vi "Lab Panel V4.91.vi"() -> ()   [LabVIEW 2013] (continued)
                          tunnel: w2787 -> [w2790 _]
                          tunnel: w2786 -> [_ w2795]
                          tunnel: w2785 -> [w2788 _]
                          frame #0 {
                            n1476 = Build Array("T-RISE") -> (w2792:string[])
                            n1477 = Build Array(w2790) -> (w2791:dbl[])
                            n1478 = TDMS Write(0:w2788, 5:"TEST PASS", 7:w2792, 9:w2791) -> (15:w2794:errorcluster)  [unwired: 2 in, 3 out]
                            n1479 = local write "data file error"(w2794) -> ()
                          }
                          frame #1 {
                            n1480 = Bundle(cluster=w2795, "STATUS"="T-RISE PASS") -> (w2797:T4)  [unwired: 2 in]
                            n1481 = local write "RESULT LAB05-2"(TRUE) -> ()
                            n1482 = local write "DISP LAB05-2"(w2797) -> ()
                          }
                        }
                      }
                      frame False {
                      }
                    }
                  }
                }
              }
            }
          }
          frame #6 {
            # "end test & close test files"
            n1483 = local read "MAIL SETTINGS"() -> (w2803:T7)
            n1484 = Unbundle(w2803) -> ("OUT SERVER ADDRESS"=w2802:string, "FROM ACCOUNT"=w2801:string)  [unwired: 5 out]
            n1485 = stacked-sequence {
              tunnel: w2813 -> [_ _ _ _ _ _ _ _ _ _]
              tunnel: w2814 -> [_ _ _ _ _ _ _ _ _ _]
              tunnel: w2812 -> [_ _ _ _ _ _ _ _ _ _]
              tunnel: w2811 -> [_ _ _ _ _ _ _ _ _ _]
              tunnel: w2810 -> [_ _ _ _ _ _ _ _ _ _]
              tunnel: w2809 -> [_ _ _ _ _ _ _ _ _ _]
              tunnel: w2808 -> [_ _ _ _ _ _ _ _ _ _]
              tunnel: w2807 -> [_ _ _ _ _ _ _ _ _ _]
              tunnel: w2806 -> [_ _ _ _ _ _ _ _ _ _]
              tunnel: w2805 -> [_ _ _ _ _ _ _ _ _ _]
              tunnel: w2802 -> [w2818 w2870 w2918 w2965 w3012 w3059 w3106 w3153 w3200 w3247]
              tunnel: w2801 -> [w2817 w2869 w2917 w2964 w3011 w3058 w3105 w3152 w3199 w3246]
              tunnel: "Mail Test File To:" -> [w2816 w2868 w2916 w2963 w3010 w3057 w3104 w3151 w3198 w3245]
              tunnel: "Mail Test Fail" -> [w2815 w2867 w2915 w2962 w3009 w3056 w3103 w3150 w3197 w3244]
              frame #0 {
                # "LAB01-1"
                n1486 = local read "DISP LAB01-1"() -> (w2822:T4)
                n1487 = local read "run lab01-1"() -> (w2819:bool)
                n1488 = local read "TDMS LAB01-1"() -> (w2820:refnum<k34>)
                n1489 = Unbundle(w2822) -> ("CYCLE"=w2823:dbl, "STATUS"=w2821:string)  [unwired: 1 out]
                n1490 = case shown="True" w2819 {
                  tunnel: w2823 -> [_ w2829]
                  tunnel: w2822 -> [_ w2831]
                  tunnel: w2821 -> [_ w2828]
                  tunnel: w2820 -> [_ w2830]
                  tunnel: w2818 -> [_ w2827]
                  tunnel: w2817 -> [_ w2826]
                  tunnel: w2816 -> [_ w2825]
                  tunnel: w2815 -> [_ w2824]
                  frame False {
                  }
                  frame True {
                    n1491 = Not Equal?(x=w2828, y="RUN") -> (x != y?=w2832:bool)
                    n1492 = Greater?(x=w2829, y=2.0) -> (0:w2834:bool)
                    n1493 = And(x=w2834, y=w2832) -> (x .and. y?=w2833:bool)
                    n1494 = case shown="True" w2833 {
                      tunnel: w2831 -> [_ w2844]
                      tunnel: w2830 -> [_ w2843]
                      tunnel: w2829 -> [_ w2842]
                      tunnel: w2828 -> [_ w2841]
                      tunnel: w2827 -> [_ w2840]
                      tunnel: w2826 -> [_ w2839]
                      tunnel: w2825 -> [_ w2838]
                      tunnel: w2824 -> [_ w2837]
                      frame False {
                      }
                      frame True {
                        n1495 = stacked-sequence {
                          tunnel: w2844 -> [w2848 _ _]
                          tunnel: w2843 -> [_ w2850 _]
                          tunnel: w2842 -> [_ _ _]
                          tunnel: w2841 -> [_ _ w2856]
                          tunnel: w2840 -> [_ _ w2855]
                          tunnel: w2839 -> [_ _ w2854]
                          tunnel: w2838 -> [_ _ w2853]
                          tunnel: w2837 -> [_ _ w2852]
                          frame #0 {
                            w2845 = FALSE
                            n1496 = local write "mail control"("END") -> ()
                            n1497 = Bundle(cluster=w2848) -> (w2847:T4)  [unwired: 3 in]
                            n1498 = local write "DISP LAB01-1"(w2847) -> ()
                            n1499 = local write "O/I  LAB01-1"(w2845) -> ()
                            n1500 = local write "run lab01-1"(w2845) -> ()
                            n1501 = local write "RUN LAB01-1"(w2845) -> ()
                          }
                          frame #1 {
                            n1502 = TDMS Close(11:w2850) -> (0:w2849:errorcluster)  [unwired: 1 in, 1 out]
                            n1503 = local write "data file error"(w2849) -> ()
                          }
                          frame #2 {
                            n1504 = stacked-sequence {
                              tunnel: "LAB01-1" -> [w2858 w2860 _]
                              tunnel: w2856 -> [_ w2866 _]
                              tunnel: w2855 -> [_ w2865 _]
                              tunnel: w2854 -> [_ w2864 _]
                              tunnel: w2853 -> [_ w2863 _]
                              tunnel: w2852 -> [_ w2862 _]
                              frame #0 {
                                n1505 = call "sub vi - defrag tdms v1.vi"("panel id"=w2858) -> ("error out"=w2857:errorcluster)  [unwired: 10 in]
                                n1506 = local write "data file error"(w2857) -> ()
                              }
                              frame #1 {
                                n1507 = Bundle("STATUS"=w2866, "OUT SERVER ADDRESS"=w2865, "FROM ACCOUNT"=w2864, "Mail Test File To:"=w2863, "Mail Test Fail"=w2862) -> (w2859:T25)  [unwired: 1 in]
                                n1508 = call "Save data file (pass-fail) v5.vi"("Input Cluster"=w2859, "panel id"=w2860) -> ("network file save error"=w2861:errorcluster)  [unwired: 8 in, 1 out]
                                n1509 = local write "data file error"(w2861) -> ()
                              }
                              frame #2 {
                              }
                            }
                          }
                        }
                      }
                    }
                  }
                }
              }
              frame #1 {
                # "LAB01-2"
                n1510 = local read "run lab01-2"() -> (w2871:bool)
                n1511 = case shown="True" w2871 {
                  tunnel: w2870 -> [_ w2875]
                  tunnel: w2869 -> [_ w2874]
                  tunnel: w2868 -> [_ w2873]
                  tunnel: w2867 -> [_ w2872]
                  frame False {
                  }
                  frame True {
                    n1512 = local read "DISP LAB01-2"() -> (w2883:T4)
                    n1513 = local read "TDMS LAB01-2"() -> (w2882:refnum<k34>)
                    n1514 = Unbundle(w2883) -> ("CYCLE"=w2877:dbl, "STATUS"=w2876:string)  [unwired: 1 out]
                    n1515 = Not Equal?(x=w2876, y="RUN") -> (x != y?=w2879:bool)
                    n1516 = Greater?(x=w2877, y=2.0) -> (0:w2880:bool)
                    n1517 = And(x=w2880, y=w2879) -> (x .and. y?=w2878:bool)
                    n1518 = case shown="True" w2878 {
                      tunnel: w2883 -> [_ w2892]
                      tunnel: w2882 -> [_ w2891]
                      tunnel: w2877 -> [_ w2890]
                      tunnel: w2876 -> [_ w2889]
                      tunnel: w2875 -> [_ w2888]
                      tunnel: w2874 -> [_ w2887]
                      tunnel: w2873 -> [_ w2886]
                      tunnel: w2872 -> [_ w2885]
                      frame False {
                      }
                      frame True {
                        n1519 = stacked-sequence {
                          tunnel: w2892 -> [w2895 _ _]
                          tunnel: w2891 -> [_ w2897 _]
                          tunnel: w2890 -> [_ _ _]
                          tunnel: w2889 -> [_ _ w2903]
                          tunnel: w2888 -> [_ _ w2902]
                          tunnel: w2887 -> [_ _ w2901]
                          tunnel: w2886 -> [_ _ w2900]
                          tunnel: w2885 -> [_ _ w2899]
                          frame #0 {
                            w2893 = FALSE
                            n1520 = local write "mail control"("END") -> ()
                            n1521 = Bundle(cluster=w2895) -> (w2896:T4)  [unwired: 3 in]
                            n1522 = local write "RUN LAB01-2"(w2893) -> ()
                            n1523 = local write "run lab01-2"(w2893) -> ()
                            n1524 = local write "O/I  LAB01-2"(w2893) -> ()
                            n1525 = local write "DISP LAB01-2"(w2896) -> ()
                          }
                          frame #1 {
                            n1526 = TDMS Close(11:w2897) -> (0:w2898:errorcluster)  [unwired: 1 in, 1 out]
                            n1527 = local write "data file error"(w2898) -> ()
                          }
                          frame #2 {
                            n1528 = stacked-sequence {
                              tunnel: "LAB01-2" -> [w2906 w2907]
                              tunnel: w2903 -> [_ w2912]
                              tunnel: w2902 -> [_ w2911]
                              tunnel: w2901 -> [_ w2910]
                              tunnel: w2900 -> [_ w2909]
                              tunnel: w2899 -> [_ w2908]
                              frame #0 {
                                n1529 = call "sub vi - defrag tdms v1.vi"("panel id"=w2906) -> ("error out"=w2905:errorcluster)  [unwired: 10 in]
                                n1530 = local write "data file error"(w2905) -> ()
                              }
                              frame #1 {
                                n1531 = Bundle("STATUS"=w2912, "OUT SERVER ADDRESS"=w2911, "FROM ACCOUNT"=w2910, "Mail Test File To:"=w2909, "Mail Test Fail"=w2908) -> (w2914:T25)  [unwired: 1 in]
                                n1532 = call "Save data file (pass-fail) v5.vi"("Input Cluster"=w2914, "panel id"=w2907) -> ("network file save error"=w2913:errorcluster)  [unwired: 8 in, 1 out]
                                n1533 = local write "data file error"(w2913) -> ()
                              }
                            }
                          }
                        }
                      }
                    }
                  }
                }
              }
              frame #2 {
                # "LAB02-1"
                n1534 = local read "run lab02-1"() -> (w2919:bool)
                n1535 = case shown="True" w2919 {
                  tunnel: w2918 -> [_ w2923]
                  tunnel: w2917 -> [_ w2922]
                  tunnel: w2916 -> [_ w2921]
                  tunnel: w2915 -> [_ w2920]
                  frame False {
                  }
                  frame True {
                    n1536 = local read "DISP LAB02-1"() -> (w2931:T4)
                    n1537 = Unbundle(w2931) -> ("CYCLE"=w2927:dbl, "STATUS"=w2924:string)  [unwired: 1 out]
                    n1538 = local read "TDMS LAB02-1"() -> (w2930:refnum<k34>)
                    n1539 = Not Equal?(x=w2924, y="RUN") -> (x != y?=w2926:bool)
                    n1540 = Greater?(x=w2927, y=2.0) -> (0:w2928:bool)
                    n1541 = And(x=w2928, y=w2926) -> (x .and. y?=w2925:bool)
                    n1542 = case shown="True" w2925 {
                      tunnel: w2931 -> [_ w2939]
                      tunnel: w2930 -> [_ w2938]
                      tunnel: w2924 -> [_ w2937]
                      tunnel: w2923 -> [_ w2936]
                      tunnel: w2922 -> [_ w2935]
                      tunnel: w2921 -> [_ w2934]
                      tunnel: w2920 -> [_ w2933]
                      frame False {
                      }
                      frame True {
                        n1543 = stacked-sequence {
                          tunnel: w2939 -> [w2942 _ _]
                          tunnel: w2938 -> [_ w2944 _]
                          tunnel: w2937 -> [_ _ w2950]
                          tunnel: w2936 -> [_ _ w2949]
                          tunnel: w2935 -> [_ _ w2948]
                          tunnel: w2934 -> [_ _ w2947]
                          tunnel: w2933 -> [_ _ w2946]
                          frame #0 {
                            w2940 = FALSE
                            n1544 = local write "mail control"("END") -> ()
                            n1545 = Bundle(cluster=w2942) -> (w2943:T4)  [unwired: 3 in]
                            n1546 = local write "O/I  LAB02-1"(w2940) -> ()
                            n1547 = local write "RUN LAB02-1"(w2940) -> ()
                            n1548 = local write "run lab02-1"(w2940) -> ()
                            n1549 = local write "DISP LAB02-1"(w2943) -> ()
                          }
                          frame #1 {
                            n1550 = TDMS Close(11:w2944) -> (0:w2945:errorcluster)  [unwired: 1 in, 1 out]
                            n1551 = local write "data file error"(w2945) -> ()
                          }
                          frame #2 {
                            n1552 = stacked-sequence {
                              tunnel: "LAB02-1" -> [w2953 w2960]
                              tunnel: w2950 -> [_ w2958]
                              tunnel: w2949 -> [_ w2957]
                              tunnel: w2948 -> [_ w2956]
                              tunnel: w2947 -> [_ w2955]
                              tunnel: w2946 -> [_ w2954]
                              frame #0 {
                                n1553 = call "sub vi - defrag tdms v1.vi"("panel id"=w2953) -> ("error out"=w2952:errorcluster)  [unwired: 10 in]
                                n1554 = local write "data file error"(w2952) -> ()
                              }
                              frame #1 {
                                n1555 = Bundle("STATUS"=w2958, "OUT SERVER ADDRESS"=w2957, "FROM ACCOUNT"=w2956, "Mail Test File To:"=w2955, "Mail Test Fail"=w2954) -> (w2959:T25)  [unwired: 1 in]
                                n1556 = call "Save data file (pass-fail) v5.vi"("Input Cluster"=w2959, "panel id"=w2960) -> ("network file save error"=w2961:errorcluster)  [unwired: 8 in, 1 out]
                                n1557 = local write "data file error"(w2961) -> ()
                              }
                            }
                          }
                        }
                      }
                    }
                  }
                }
              }
              frame #3 {
                # "LAB02-2"
                n1558 = local read "run lab02-2"() -> (w2966:bool)
                n1559 = case shown="True" w2966 {
                  tunnel: w2965 -> [_ w2970]
                  tunnel: w2964 -> [_ w2969]
                  tunnel: w2963 -> [_ w2968]
                  tunnel: w2962 -> [_ w2967]
                  frame False {
                  }
                  frame True {
                    n1560 = local read "DISP LAB02-2"() -> (w2978:T4)
                    n1561 = local read "TDMS LAB02-2"() -> (w2977:refnum<k34>)
                    n1562 = Unbundle(w2978) -> ("CYCLE"=w2974:dbl, "STATUS"=w2971:string)  [unwired: 1 out]
                    n1563 = Not Equal?(x=w2971, y="RUN") -> (x != y?=w2973:bool)
                    n1564 = Greater?(x=w2974, y=2.0) -> (0:w2975:bool)
                    n1565 = And(x=w2975, y=w2973) -> (x .and. y?=w2972:bool)
                    n1566 = case shown="True" w2972 {
                      tunnel: w2978 -> [_ w2986]
                      tunnel: w2977 -> [_ w2985]
                      tunnel: w2971 -> [_ w2984]
                      tunnel: w2970 -> [_ w2983]
                      tunnel: w2969 -> [_ w2982]
                      tunnel: w2968 -> [_ w2981]
                      tunnel: w2967 -> [_ w2980]
                      frame False {
                      }
                      frame True {
                        n1567 = stacked-sequence {
                          tunnel: w2986 -> [w2989 _ _]
                          tunnel: w2985 -> [_ w2991 _]
                          tunnel: w2984 -> [_ _ w2997]
                          tunnel: w2983 -> [_ _ w2996]
                          tunnel: w2982 -> [_ _ w2995]
                          tunnel: w2981 -> [_ _ w2994]
                          tunnel: w2980 -> [_ _ w2993]
                          frame #0 {
                            w2987 = FALSE
                            n1568 = local write "mail control"("END") -> ()
                            n1569 = Bundle(cluster=w2989) -> (w2990:T4)  [unwired: 3 in]
                            n1570 = local write "O/I  LAB02-2"(w2987) -> ()
                            n1571 = local write "run lab02-2"(w2987) -> ()
                            n1572 = local write "RUN LAB02-2"(w2987) -> ()
                            n1573 = local write "DISP LAB02-2"(w2990) -> ()
                          }
                          frame #1 {
                            n1574 = TDMS Close(11:w2991) -> (0:w2992:errorcluster)  [unwired: 1 in, 1 out]
                            n1575 = local write "data file error"(w2992) -> ()
                          }
                          frame #2 {
                            n1576 = stacked-sequence {
                              tunnel: "LAB02-2" -> [w3000 w3006]
                              tunnel: w2997 -> [_ w3005]
                              tunnel: w2996 -> [_ w3004]
                              tunnel: w2995 -> [_ w3003]
                              tunnel: w2994 -> [_ w3002]
                              tunnel: w2993 -> [_ w3001]
                              frame #0 {
                                n1577 = call "sub vi - defrag tdms v1.vi"("panel id"=w3000) -> ("error out"=w2999:errorcluster)  [unwired: 10 in]
                                n1578 = local write "data file error"(w2999) -> ()
                              }
                              frame #1 {
                                n1579 = Bundle("STATUS"=w3005, "OUT SERVER ADDRESS"=w3004, "FROM ACCOUNT"=w3003, "Mail Test File To:"=w3002, "Mail Test Fail"=w3001) -> (w3008:T25)  [unwired: 1 in]
                                n1580 = call "Save data file (pass-fail) v5.vi"("Input Cluster"=w3008, "panel id"=w3006) -> ("network file save error"=w3007:errorcluster)  [unwired: 8 in, 1 out]
                                n1581 = local write "data file error"(w3007) -> ()
                              }
                            }
                          }
                        }
                      }
                    }
                  }
                }
              }
              frame #4 {
                # "LAB03-1"
                n1582 = local read "run lab03-1"() -> (w3013:bool)
                n1583 = case shown="True" w3013 {
                  tunnel: w3012 -> [_ w3017]
                  tunnel: w3011 -> [_ w3016]
                  tunnel: w3010 -> [_ w3015]
                  tunnel: w3009 -> [_ w3014]
                  frame False {
                  }
                  frame True {
                    n1584 = local read "DISP LAB03-1"() -> (w3025:T4)
                    n1585 = local read "TDMS LAB03-1"() -> (w3024:refnum<k34>)
                    n1586 = Unbundle(w3025) -> ("CYCLE"=w3021:dbl, "STATUS"=w3018:string)  [unwired: 1 out]
                    n1587 = Not Equal?(x=w3018, y="RUN") -> (x != y?=w3020:bool)
                    n1588 = Greater?(x=w3021, y=2.0) -> (0:w3022:bool)
                    n1589 = And(x=w3022, y=w3020) -> (x .and. y?=w3019:bool)
                    n1590 = case shown="True" w3019 {
                      tunnel: w3025 -> [_ w3033]
                      tunnel: w3024 -> [_ w3032]
                      tunnel: w3018 -> [_ w3031]
                      tunnel: w3017 -> [_ w3030]
                      tunnel: w3016 -> [_ w3029]
                      tunnel: w3015 -> [_ w3028]
                      tunnel: w3014 -> [_ w3027]
                      frame False {
                      }
                      frame True {
                        n1591 = stacked-sequence {
                          tunnel: w3033 -> [w3036 _ _]
                          tunnel: w3032 -> [_ w3038 _]
                          tunnel: w3031 -> [_ _ w3044]
                          tunnel: w3030 -> [_ _ w3043]
                          tunnel: w3029 -> [_ _ w3042]
                          tunnel: w3028 -> [_ _ w3041]
                          tunnel: w3027 -> [_ _ w3040]
                          frame #0 {
                            w3034 = FALSE
                            n1592 = local write "mail control"("END") -> ()
                            n1593 = Bundle(cluster=w3036) -> (w3037:T4)  [unwired: 3 in]
                            n1594 = local write "O/I  LAB03-1"(w3034) -> ()
                            n1595 = local write "run lab03-1"(w3034) -> ()
                            n1596 = local write "RUN LAB03-1"(w3034) -> ()
                            n1597 = local write "DISP LAB03-1"(w3037) -> ()
                          }
                          frame #1 {
                            n1598 = TDMS Close(11:w3038) -> (0:w3039:errorcluster)  [unwired: 1 in, 1 out]
                            n1599 = local write "data file error"(w3039) -> ()
                          }
                          frame #2 {
                            n1600 = stacked-sequence {
                              tunnel: "LAB03-1" -> [w3047 w3053]
                              tunnel: w3044 -> [_ w3052]
                              tunnel: w3043 -> [_ w3051]
                              tunnel: w3042 -> [_ w3050]
                              tunnel: w3041 -> [_ w3049]
                              tunnel: w3040 -> [_ w3048]
                              frame #0 {
                                n1601 = call "sub vi - defrag tdms v1.vi"("panel id"=w3047) -> ("error out"=w3046:errorcluster)  [unwired: 10 in]
                                n1602 = local write "data file error"(w3046) -> ()
                              }
                              frame #1 {
                                n1603 = Bundle("STATUS"=w3052, "OUT SERVER ADDRESS"=w3051, "FROM ACCOUNT"=w3050, "Mail Test File To:"=w3049, "Mail Test Fail"=w3048) -> (w3055:T25)  [unwired: 1 in]
                                n1604 = call "Save data file (pass-fail) v5.vi"("Input Cluster"=w3055, "panel id"=w3053) -> ("network file save error"=w3054:errorcluster)  [unwired: 8 in, 1 out]
                                n1605 = local write "data file error"(w3054) -> ()
                              }
                            }
                          }
                        }
                      }
                    }
                  }
                }
              }
              frame #5 {
                # "LAB03-2"
                n1606 = local read "run lab03-2"() -> (w3060:bool)
                n1607 = case shown="True" w3060 {
                  tunnel: w3059 -> [_ w3064]
                  tunnel: w3058 -> [_ w3063]
                  tunnel: w3057 -> [_ w3062]
                  tunnel: w3056 -> [_ w3061]
                  frame False {
                  }
                  frame True {
                    n1608 = local read "DISP LAB03-2"() -> (w3072:T4)
                    n1609 = Unbundle(w3072) -> ("CYCLE"=w3068:dbl, "STATUS"=w3065:string)  [unwired: 1 out]
                    n1610 = local read "TDMS LAB03-2"() -> (w3071:refnum<k34>)
                    n1611 = Not Equal?(x=w3065, y="RUN") -> (x != y?=w3067:bool)
                    n1612 = Greater?(x=w3068, y=2.0) -> (0:w3069:bool)
                    n1613 = And(x=w3069, y=w3067) -> (x .and. y?=w3066:bool)
                    n1614 = case shown="True" w3066 {
                      tunnel: w3072 -> [_ w3080]
                      tunnel: w3071 -> [_ w3079]
                      tunnel: w3065 -> [_ w3078]
                      tunnel: w3064 -> [_ w3077]
                      tunnel: w3063 -> [_ w3076]
                      tunnel: w3062 -> [_ w3075]
                      tunnel: w3061 -> [_ w3074]
                      frame False {
                      }
                      frame True {
                        n1615 = stacked-sequence {
                          tunnel: w3080 -> [w3083 _ _]
                          tunnel: w3079 -> [_ w3085 _]
                          tunnel: w3078 -> [_ _ w3091]
                          tunnel: w3077 -> [_ _ w3090]
                          tunnel: w3076 -> [_ _ w3089]
                          tunnel: w3075 -> [_ _ w3088]
                          tunnel: w3074 -> [_ _ w3087]
                          frame #0 {
                            w3081 = FALSE
                            n1616 = local write "mail control"("END") -> ()
                            n1617 = Bundle(cluster=w3083) -> (w3084:T4)  [unwired: 3 in]
                            n1618 = local write "RUN LAB03-2"(w3081) -> ()
                            n1619 = local write "O/I  LAB03-2"(w3081) -> ()
                            n1620 = local write "DISP LAB03-2"(w3084) -> ()
                            n1621 = local write "run lab03-2"(w3081) -> ()
                          }
                          frame #1 {
                            n1622 = TDMS Close(11:w3085) -> (0:w3086:errorcluster)  [unwired: 1 in, 1 out]
                            n1623 = local write "data file error"(w3086) -> ()
                          }
                          frame #2 {
                            n1624 = stacked-sequence {
                              tunnel: "LAB03-2" -> [w3094 w3095]
                              tunnel: w3091 -> [_ w3100]
                              tunnel: w3090 -> [_ w3099]
                              tunnel: w3089 -> [_ w3098]
                              tunnel: w3088 -> [_ w3097]
                              tunnel: w3087 -> [_ w3096]
                              frame #0 {
                                n1625 = call "sub vi - defrag tdms v1.vi"("panel id"=w3094) -> ("error out"=w3093:errorcluster)  [unwired: 10 in]
                                n1626 = local write "data file error"(w3093) -> ()
                              }
                              frame #1 {
                                n1627 = Bundle("STATUS"=w3100, "OUT SERVER ADDRESS"=w3099, "FROM ACCOUNT"=w3098, "Mail Test File To:"=w3097, "Mail Test Fail"=w3096) -> (w3102:T25)  [unwired: 1 in]
                                n1628 = call "Save data file (pass-fail) v5.vi"("Input Cluster"=w3102, "panel id"=w3095) -> ("network file save error"=w3101:errorcluster)  [unwired: 8 in, 1 out]
                                n1629 = local write "data file error"(w3101) -> ()
                              }
                            }
                          }
                        }
                      }
                    }
                  }
                }
              }
              frame #6 {
                # "LAB04-1"
                n1630 = local read "run lab04-1"() -> (w3107:bool)
                n1631 = case shown="True" w3107 {
                  tunnel: w3106 -> [_ w3111]
                  tunnel: w3105 -> [_ w3110]
                  tunnel: w3104 -> [_ w3109]
                  tunnel: w3103 -> [_ w3108]
                  frame False {
                  }
                  frame True {
                    n1632 = local read "DISP LAB04-1"() -> (w3119:T4)
                    n1633 = Unbundle(w3119) -> ("CYCLE"=w3115:dbl, "STATUS"=w3112:string)  [unwired: 1 out]
                    n1634 = local read "TDMS LAB04-1"() -> (w3118:refnum<k34>)
                    n1635 = Not Equal?(x=w3112, y="RUN") -> (x != y?=w3114:bool)
                    n1636 = Greater?(x=w3115, y=2.0) -> (0:w3116:bool)
                    n1637 = And(x=w3116, y=w3114) -> (x .and. y?=w3113:bool)
                    n1638 = case shown="True" w3113 {
                      tunnel: w3119 -> [_ w3127]
                      tunnel: w3118 -> [_ w3126]
                      tunnel: w3112 -> [_ w3125]
                      tunnel: w3111 -> [_ w3124]
                      tunnel: w3110 -> [_ w3123]
                      tunnel: w3109 -> [_ w3122]
                      tunnel: w3108 -> [_ w3121]
                      frame False {
                      }
                      frame True {
                        n1639 = stacked-sequence {
                          tunnel: w3127 -> [w3130 _ _]
                          tunnel: w3126 -> [_ w3132 _]
                          tunnel: w3125 -> [_ _ w3138]
                          tunnel: w3124 -> [_ _ w3137]
                          tunnel: w3123 -> [_ _ w3136]
                          tunnel: w3122 -> [_ _ w3135]
                          tunnel: w3121 -> [_ _ w3134]
                          frame #0 {
                            w3128 = FALSE
                            n1640 = local write "mail control"("END") -> ()
                            n1641 = Bundle(cluster=w3130) -> (w3131:T4)  [unwired: 3 in]
                            n1642 = local write "RUN LAB04-1"(w3128) -> ()
                            n1643 = local write "O/I  LAB04-1"(w3128) -> ()
                            n1644 = local write "run lab04-1"(w3128) -> ()
                            n1645 = local write "DISP LAB04-1"(w3131) -> ()
                          }
                          frame #1 {
                            n1646 = TDMS Close(11:w3132) -> (0:w3133:errorcluster)  [unwired: 1 in, 1 out]
                            n1647 = local write "data file error"(w3133) -> ()
                          }
                          frame #2 {
                            n1648 = stacked-sequence {
                              tunnel: "LAB04-1" -> [w3141 w3142]
                              tunnel: w3138 -> [_ w3147]
                              tunnel: w3137 -> [_ w3146]
                              tunnel: w3136 -> [_ w3145]
                              tunnel: w3135 -> [_ w3144]
                              tunnel: w3134 -> [_ w3143]
                              frame #0 {
                                n1649 = call "sub vi - defrag tdms v1.vi"("panel id"=w3141) -> ("error out"=w3140:errorcluster)  [unwired: 10 in]
                                n1650 = local write "data file error"(w3140) -> ()
                              }
                              frame #1 {
                                n1651 = Bundle("STATUS"=w3147, "OUT SERVER ADDRESS"=w3146, "FROM ACCOUNT"=w3145, "Mail Test File To:"=w3144, "Mail Test Fail"=w3143) -> (w3149:T25)  [unwired: 1 in]
                                n1652 = call "Save data file (pass-fail) v5.vi"("Input Cluster"=w3149, "panel id"=w3142) -> ("network file save error"=w3148:errorcluster)  [unwired: 8 in, 1 out]
                                n1653 = local write "data file error"(w3148) -> ()
                              }
                            }
                          }
                        }
                      }
                    }
                  }
                }
              }
              frame #7 {
                # "LAB04-2"
                n1654 = local read "run lab04-2"() -> (w3154:bool)
                n1655 = case shown="True" w3154 {
                  tunnel: w3153 -> [_ w3158]
                  tunnel: w3152 -> [_ w3157]
                  tunnel: w3151 -> [_ w3156]
                  tunnel: w3150 -> [_ w3155]
                  frame False {
                  }
                  frame True {
                    n1656 = local read "DISP LAB04-2"() -> (w3166:T4)
                    n1657 = Unbundle(w3166) -> ("CYCLE"=w3162:dbl, "STATUS"=w3159:string)  [unwired: 1 out]
                    n1658 = Not Equal?(x=w3159, y="RUN") -> (x != y?=w3161:bool)
                    n1659 = local read "TDMS LAB04-2"() -> (w3165:refnum<k34>)
                    n1660 = Greater?(x=w3162, y=2.0) -> (0:w3163:bool)
                    n1661 = And(x=w3163, y=w3161) -> (x .and. y?=w3160:bool)
                    n1662 = case shown="True" w3160 {
                      tunnel: w3166 -> [_ w3174]
                      tunnel: w3165 -> [_ w3173]
                      tunnel: w3159 -> [_ w3172]
                      tunnel: w3158 -> [_ w3171]
                      tunnel: w3157 -> [_ w3170]
                      tunnel: w3156 -> [_ w3169]
                      tunnel: w3155 -> [_ w3168]
                      frame False {
                      }
                      frame True {
                        n1663 = stacked-sequence {
                          tunnel: w3174 -> [w3177 _ _]
                          tunnel: w3173 -> [_ w3179 _]
                          tunnel: w3172 -> [_ _ w3185]
                          tunnel: w3171 -> [_ _ w3184]
                          tunnel: w3170 -> [_ _ w3183]
                          tunnel: w3169 -> [_ _ w3182]
                          tunnel: w3168 -> [_ _ w3181]
                          frame #0 {
                            w3175 = FALSE
                            n1664 = local write "mail control"("END") -> ()
                            n1665 = Bundle(cluster=w3177) -> (w3178:T4)  [unwired: 3 in]
                            n1666 = local write "O/I  LAB04-2"(w3175) -> ()
                            n1667 = local write "RUN LAB04-2"(w3175) -> ()
                            n1668 = local write "run lab04-2"(w3175) -> ()
                            n1669 = local write "DISP LAB04-2"(w3178) -> ()
                          }
                          frame #1 {
                            n1670 = TDMS Close(11:w3179) -> (0:w3180:errorcluster)  [unwired: 1 in, 1 out]
                            n1671 = local write "data file error"(w3180) -> ()
                          }
                          frame #2 {
                            n1672 = stacked-sequence {
                              tunnel: "LAB04-2" -> [w3188 w3189]
                              tunnel: w3185 -> [_ w3194]
                              tunnel: w3184 -> [_ w3193]
                              tunnel: w3183 -> [_ w3192]
                              tunnel: w3182 -> [_ w3191]
                              tunnel: w3181 -> [_ w3190]
                              frame #0 {
                                n1673 = call "sub vi - defrag tdms v1.vi"("panel id"=w3188) -> ("error out"=w3187:errorcluster)  [unwired: 10 in]
                                n1674 = local write "data file error"(w3187) -> ()
                              }
                              frame #1 {
                                n1675 = Bundle("STATUS"=w3194, "OUT SERVER ADDRESS"=w3193, "FROM ACCOUNT"=w3192, "Mail Test File To:"=w3191, "Mail Test Fail"=w3190) -> (w3196:T25)  [unwired: 1 in]
                                n1676 = call "Save data file (pass-fail) v5.vi"("Input Cluster"=w3196, "panel id"=w3189) -> ("network file save error"=w3195:errorcluster)  [unwired: 8 in, 1 out]
                                n1677 = local write "data file error"(w3195) -> ()
                              }
                            }
                          }
                        }
                      }
                    }
                  }
                }
              }
              frame #8 {
                # "LAB05-1"
                n1678 = local read "run lab05-1"() -> (w3201:bool)
                n1679 = case shown="True" w3201 {
                  tunnel: w3200 -> [_ w3205]
                  tunnel: w3199 -> [_ w3204]
                  tunnel: w3198 -> [_ w3203]
                  tunnel: w3197 -> [_ w3202]
                  frame False {
                  }
                  frame True {
                    n1680 = local read "DISP LAB05-1"() -> (w3213:T4)
                    n1681 = Unbundle(w3213) -> ("CYCLE"=w3209:dbl, "STATUS"=w3206:string)  [unwired: 1 out]
                    n1682 = Not Equal?(x=w3206, y="RUN") -> (x != y?=w3208:bool)
                    n1683 = local read "TDMS LAB05-1"() -> (w3212:refnum<k34>)
                    n1684 = Greater?(x=w3209, y=2.0) -> (0:w3210:bool)
                    n1685 = And(x=w3210, y=w3208) -> (x .and. y?=w3207:bool)
                    n1686 = case shown="True" w3207 {
                      tunnel: w3213 -> [_ w3221]
                      tunnel: w3212 -> [_ w3220]
                      tunnel: w3206 -> [_ w3219]
                      tunnel: w3205 -> [_ w3218]
                      tunnel: w3204 -> [_ w3217]
                      tunnel: w3203 -> [_ w3216]
                      tunnel: w3202 -> [_ w3215]
                      frame False {
                      }
                      frame True {
                        n1687 = stacked-sequence {
                          tunnel: w3221 -> [w3224 _ _]
                          tunnel: w3220 -> [_ w3226 _]
                          tunnel: w3219 -> [_ _ w3232]
                          tunnel: w3218 -> [_ _ w3231]
                          tunnel: w3217 -> [_ _ w3230]
                          tunnel: w3216 -> [_ _ w3229]
                          tunnel: w3215 -> [_ _ w3228]
                          frame #0 {
                            w3222 = FALSE
                            n1688 = local write "mail control"("END") -> ()
                            n1689 = Bundle(cluster=w3224) -> (w3225:T4)  [unwired: 3 in]
                            n1690 = local write "O/I  LAB05-1"(w3222) -> ()
                            n1691 = local write "RUN LAB05-1"(w3222) -> ()
                            n1692 = local write "run lab05-1"(w3222) -> ()
                            n1693 = local write "DISP LAB05-1"(w3225) -> ()
                          }
                          frame #1 {
                            n1694 = TDMS Close(11:w3226) -> (0:w3227:errorcluster)  [unwired: 1 in, 1 out]
                            n1695 = local write "data file error"(w3227) -> ()
                          }
                          frame #2 {
                            n1696 = stacked-sequence {
                              tunnel: "LAB05-1" -> [w3235 w3241]
                              tunnel: w3232 -> [_ w3240]
                              tunnel: w3231 -> [_ w3239]
                              tunnel: w3230 -> [_ w3238]
                              tunnel: w3229 -> [_ w3237]
                              tunnel: w3228 -> [_ w3236]
                              frame #0 {
                                n1697 = call "sub vi - defrag tdms v1.vi"("panel id"=w3235) -> ("error out"=w3234:errorcluster)  [unwired: 10 in]
                                n1698 = local write "data file error"(w3234) -> ()
                              }
                              frame #1 {
                                n1699 = Bundle("STATUS"=w3240, "OUT SERVER ADDRESS"=w3239, "FROM ACCOUNT"=w3238, "Mail Test File To:"=w3237, "Mail Test Fail"=w3236) -> (w3243:T25)  [unwired: 1 in]
                                n1700 = call "Save data file (pass-fail) v5.vi"("Input Cluster"=w3243, "panel id"=w3241) -> ("network file save error"=w3242:errorcluster)  [unwired: 8 in, 1 out]
                                n1701 = local write "data file error"(w3242) -> ()
                              }
                            }
                          }
                        }
                      }
                    }
                  }
                }
              }
              frame #9 {
                # "LAB05-2"
                n1702 = local read "run lab05-2"() -> (w3248:bool)
                n1703 = case shown="True" w3248 {
                  tunnel: w3247 -> [_ w3252]
                  tunnel: w3246 -> [_ w3251]
                  tunnel: w3245 -> [_ w3250]
                  tunnel: w3244 -> [_ w3249]
                  frame False {
                  }
                  frame True {
                    n1704 = local read "DISP LAB05-2"() -> (w3260:T4)
                    n1705 = Unbundle(w3260) -> ("CYCLE"=w3256:dbl, "STATUS"=w3253:string)  [unwired: 1 out]
                    n1706 = Not Equal?(x=w3253, y="RUN") -> (x != y?=w3255:bool)
                    n1707 = local read "TDMS LAB05-2"() -> (w3259:refnum<k34>)
                    n1708 = Greater?(x=w3256, y=2.0) -> (0:w3257:bool)
                    n1709 = And(x=w3257, y=w3255) -> (x .and. y?=w3254:bool)
                    n1710 = case shown="True" w3254 {
                      tunnel: w3260 -> [_ w3268]
                      tunnel: w3259 -> [_ w3267]
                      tunnel: w3253 -> [_ w3266]
                      tunnel: w3252 -> [_ w3265]
                      tunnel: w3251 -> [_ w3264]
                      tunnel: w3250 -> [_ w3263]
                      tunnel: w3249 -> [_ w3262]
                      frame False {
                      }
                      frame True {
                        n1711 = stacked-sequence {
                          tunnel: w3268 -> [w3271 _ _]
                          tunnel: w3267 -> [_ w3273 _]
                          tunnel: w3266 -> [_ _ w3279]
                          tunnel: w3265 -> [_ _ w3278]
                          tunnel: w3264 -> [_ _ w3277]
                          tunnel: w3263 -> [_ _ w3276]
                          tunnel: w3262 -> [_ _ w3275]
                          frame #0 {
                            w3269 = FALSE
                            n1712 = local write "mail control"("END") -> ()
                            n1713 = Bundle(cluster=w3271) -> (w3272:T4)  [unwired: 3 in]
                            n1714 = local write "RUN LAB05-2"(w3269) -> ()
                            n1715 = local write "O/I  LAB05-2"(w3269) -> ()
                            n1716 = local write "run lab05-2"(w3269) -> ()
                            n1717 = local write "DISP LAB05-2"(w3272) -> ()
                          }
                          frame #1 {
                            n1718 = TDMS Close(11:w3273) -> (0:w3274:errorcluster)  [unwired: 1 in, 1 out]
                            n1719 = local write "data file error"(w3274) -> ()
                          }
                          frame #2 {
                            n1720 = stacked-sequence {
                              tunnel: "LAB05-2" -> [w3282 w3288]
                              tunnel: w3279 -> [_ w3287]
                              tunnel: w3278 -> [_ w3286]
                              tunnel: w3277 -> [_ w3285]
                              tunnel: w3276 -> [_ w3284]
                              tunnel: w3275 -> [_ w3283]
                              frame #0 {
                                n1721 = call "sub vi - defrag tdms v1.vi"("panel id"=w3282) -> ("error out"=w3281:errorcluster)  [unwired: 10 in]
                                n1722 = local write "data file error"(w3281) -> ()
                              }
                              frame #1 {
                                n1723 = Bundle("STATUS"=w3287, "OUT SERVER ADDRESS"=w3286, "FROM ACCOUNT"=w3285, "Mail Test File To:"=w3284, "Mail Test Fail"=w3283) -> (w3290:T25)  [unwired: 1 in]
                                n1724 = call "Save data file (pass-fail) v5.vi"("Input Cluster"=w3290, "panel id"=w3288) -> ("network file save error"=w3289:errorcluster)  [unwired: 8 in, 1 out]
                                n1725 = local write "data file error"(w3289) -> ()
                              }
                            }
                          }
                        }
                      }
                    }
                  }
                }
              }
            }
            n1726 = local read "Network Directory"() -> (w2804:path)
            n1727 = global write "Global 1.vi" "Network Drive"(w2804) -> ()
          }
          frame #7 {
            # "disable functions"
            n1728 = stacked-sequence {
              tunnel: w3300 -> [w3314 _ w3371]
              tunnel: w3299 -> [w3309 _ w3370]
              tunnel: w3298 -> [w3308 _ w3369]
              tunnel: w3297 -> [w3306 _ w3368]
              tunnel: w3296 -> [w3307 _ w3367]
              tunnel: w3295 -> [_ w3331 w3366]
              tunnel: w3294 -> [_ w3332 w3365]
              tunnel: w3293 -> [_ w3333 w3364]
              tunnel: w3292 -> [_ w3334 w3363]
              tunnel: w3291 -> [_ w3335 w3362]
              frame #0 {
                n1729 = Select(t=2, s=w3306, f=0) -> (s? t:f=w3302:i32)
                n1730 = Select(t=2, s=w3308, f=0) -> (s? t:f=w3303:i32)
                n1731 = Select(t=2, s=w3307, f=0) -> (s? t:f=w3301:i32)
                n1732 = Select(t=2, s=w3314, f=0) -> (s? t:f=w3305:i32)
                n1733 = Select(t=2, s=w3309, f=0) -> (s? t:f=w3304:i32)
                n1734 = property on="SELECT LAB02-2" class="RadioBtnsControl (strict)"("DisabledEnum"=w3302) -> ()  [unwired: 2 in, 2 out]
                n1735 = property on="SELECT LAB02-1" class="RadioBtnsControl (strict)"("DisabledEnum"=w3303) -> ()  [unwired: 2 in, 2 out]
                n1736 = property on="SELECT LAB03-1" class="RadioBtnsControl (strict)"("DisabledEnum"=w3301) -> ()  [unwired: 2 in, 2 out]
                n1737 = property on="SELECT LAB01-1" class="RadioBtnsControl (strict)"("DisabledEnum"=w3305) -> ()  [unwired: 2 in, 2 out]
                n1738 = property on="SELECT LAB01-2" class="RadioBtnsControl (strict)"("DisabledEnum"=w3304) -> ()  [unwired: 2 in, 2 out]
                n1739 = Not(x=w3314) -> (.not. x?=w3315:bool)
                n1740 = property on="RESULT LAB01-1" class="Bool (strict)"("Visible"=w3315) -> ()  [unwired: 2 in, 2 out]
                n1741 = Not(x=w3309) -> (.not. x?=w3313:bool)
                n1742 = Not(x=w3308) -> (.not. x?=w3312:bool)
                n1743 = Not(x=w3306) -> (.not. x?=w3311:bool)
                n1744 = property on="RESULT LAB01-2" class="Bool (strict)"("Visible"=w3313) -> ()  [unwired: 2 in, 2 out]
                n1745 = Not(x=w3307) -> (.not. x?=w3310:bool)
                n1746 = property on="RESULT LAB02-1" class="Bool (strict)"("Visible"=w3312) -> ()  [unwired: 2 in, 2 out]
                n1747 = property on="RESULT LAB02-2" class="Bool (strict)"("Visible"=w3311) -> ()  [unwired: 2 in, 2 out]
                n1748 = property on="RESULT LAB03-1" class="Bool (strict)"("Visible"=w3310) -> ()  [unwired: 2 in, 2 out]
                n1749 = property on="SET LAB01-1" class="Clust (strict)"("DisabledEnum"=w3305) -> ()  [unwired: 2 in, 2 out]
                n1750 = property on="SET LAB01-2" class="Clust (strict)"("DisabledEnum"=w3304) -> ()  [unwired: 2 in, 2 out]
                n1751 = property on="SET LAB02-1" class="Clust (strict)"("DisabledEnum"=w3303) -> ()  [unwired: 2 in, 2 out]
                n1752 = property on="SET LAB02-2" class="Clust (strict)"("DisabledEnum"=w3302) -> ()  [unwired: 2 in, 2 out]
                n1753 = property on="SET LAB03-1" class="Clust (strict)"("DisabledEnum"=w3301) -> ()  [unwired: 2 in, 2 out]
                n1754 = property on="O/I  LAB01-1" class="Bool (strict)"("DisabledEnum"=w3305) -> ()  [unwired: 2 in, 2 out]
                n1755 = property on="O/I  LAB01-2" class="Bool (strict)"("DisabledEnum"=w3304) -> ()  [unwired: 2 in, 2 out]
                n1756 = property on="O/I  LAB02-1" class="Bool (strict)"("DisabledEnum"=w3303) -> ()  [unwired: 2 in, 2 out]
                n1757 = property on="O/I  LAB02-2" class="Bool (strict)"("DisabledEnum"=w3302) -> ()  [unwired: 2 in, 2 out]
                n1758 = property on="O/I  LAB03-1" class="Bool (strict)"("DisabledEnum"=w3301) -> ()  [unwired: 2 in, 2 out]
              }
              frame #1 {
                n1759 = Select(t=2, s=w3335, f=0) -> (s? t:f=w3326:i32)
                n1760 = Select(t=2, s=w3334, f=0) -> (s? t:f=w3327:i32)
                n1761 = Select(t=2, s=w3331, f=0) -> (s? t:f=w3330:i32)
                n1762 = Select(t=2, s=w3332, f=0) -> (s? t:f=w3329:i32)
                n1763 = Select(t=2, s=w3333, f=0) -> (s? t:f=w3328:i32)
                n1764 = property on="SELECT LAB05-2" class="RadioBtnsControl (strict)"("DisabledEnum"=w3326) -> ()  [unwired: 2 in, 2 out]
                n1765 = property on="SELECT LAB05-1" class="RadioBtnsControl (strict)"("DisabledEnum"=w3327) -> ()  [unwired: 2 in, 2 out]
                n1766 = property on="SELECT LAB03-2" class="RadioBtnsControl (strict)"("DisabledEnum"=w3330) -> ()  [unwired: 2 in, 2 out]
                n1767 = property on="SELECT LAB04-1" class="RadioBtnsControl (strict)"("DisabledEnum"=w3329) -> ()  [unwired: 2 in, 2 out]
                n1768 = property on="SELECT LAB04-2" class="RadioBtnsControl (strict)"("DisabledEnum"=w3328) -> ()  [unwired: 2 in, 2 out]
                n1769 = property on="SET LAB05-2" class="Clust (strict)"("DisabledEnum"=w3326) -> ()  [unwired: 2 in, 2 out]
                n1770 = property on="SET LAB05-1" class="Clust (strict)"("DisabledEnum"=w3327) -> ()  [unwired: 2 in, 2 out]
